vi "Alarma.vi"() -> ()   [LabVIEW 2020]
panel:
  out "Resultado":dbl
  out "String":string
  out "Boolean":bool
  out "Tank":dbl(slide) scale=0.0..100.0
  in  "Alarma":dbl(slide) scale=0.0..100.0
  in  "Temperatura":dbl(slide) scale=0.0..100.0
  # "Indicador de Alarma"
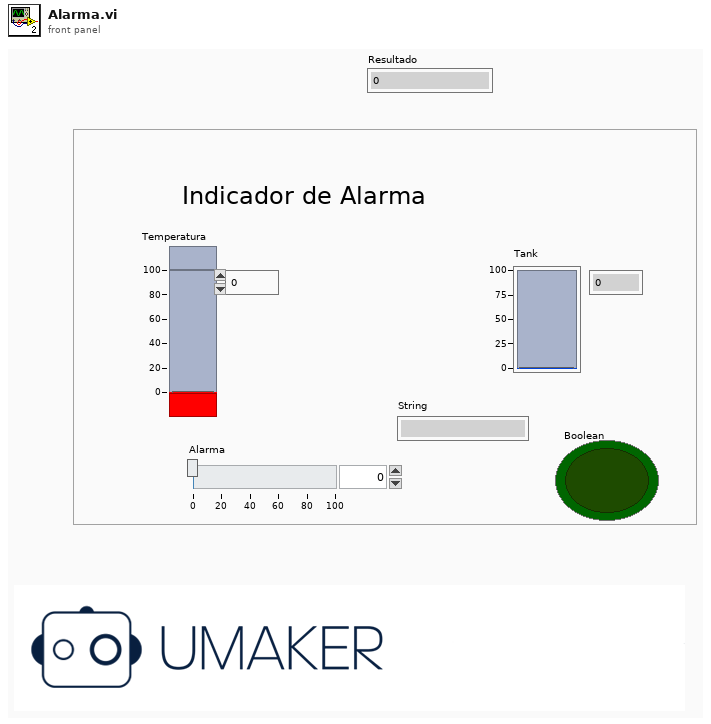
[diagram p1: front panel]
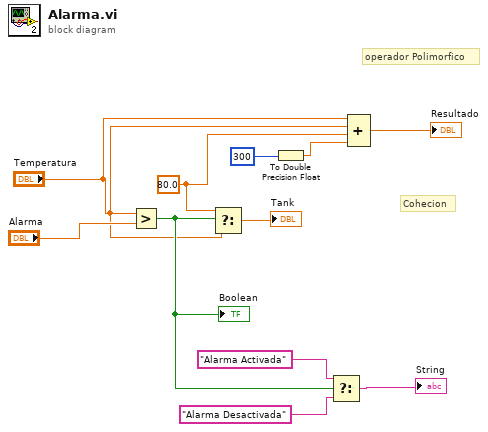
[diagram p0: block diagram]
diagram:
  w4 = 80.0
  # "Cohecion"
  # "operador Polimorfico"
  n1 = Greater?(x="Temperatura", y="Alarma") -> (0:w9:bool)
  "Boolean" <- w9
  n2 = Select(t=w4, s=w9, f="Temperatura") -> (s? t:f=→"Tank":dbl)
  n3 = To Double Precision Float(number=300) -> (double precision float=w1:dbl)
  n4 = Select(t="Alarma Activada", s=w9, f="Alarma Desactivada") -> (s? t:f=→"String":string)
  n5 = Compound Arithmetic op=ADD("Temperatura", "Temperatura", w4, w1) -> (→"Resultado":dbl)
